vi "FTW-Listener-Destroy.vi"(0 "Gmsg_Listener In":refnum<class "FTW-Listener.lvclass">, 11 "error in":errorcluster) -> (15 "error out":errorcluster)   [LabVIEW 2013, in "FTW-Listener.lvclass"]
uses:
  FTW-Listener.lvclass
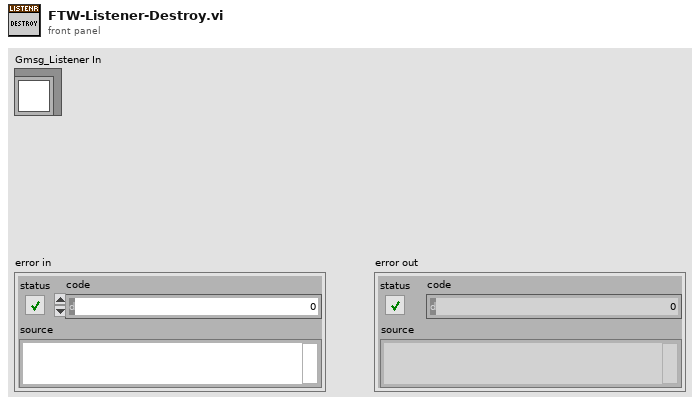
[diagram p1: front panel]
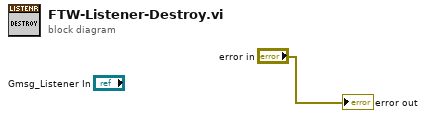
[diagram p0: block diagram]
diagram:
  "error out" <- "error in"
